vi "add_test.vi"() -> ()   [LabVIEW 2018]
panel:
  in  "Input Parameters":string
  out "Current Pressure [Torr]":dbl
  out "Average Pressure [Torr]":dbl
  out "Average Press.  < 2.2E-4 Torr?":bool
  in  "Run Scan?":bool
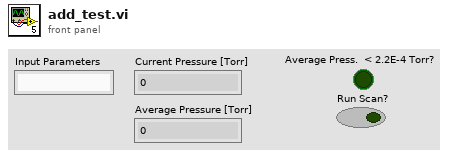
[diagram p1: front panel]
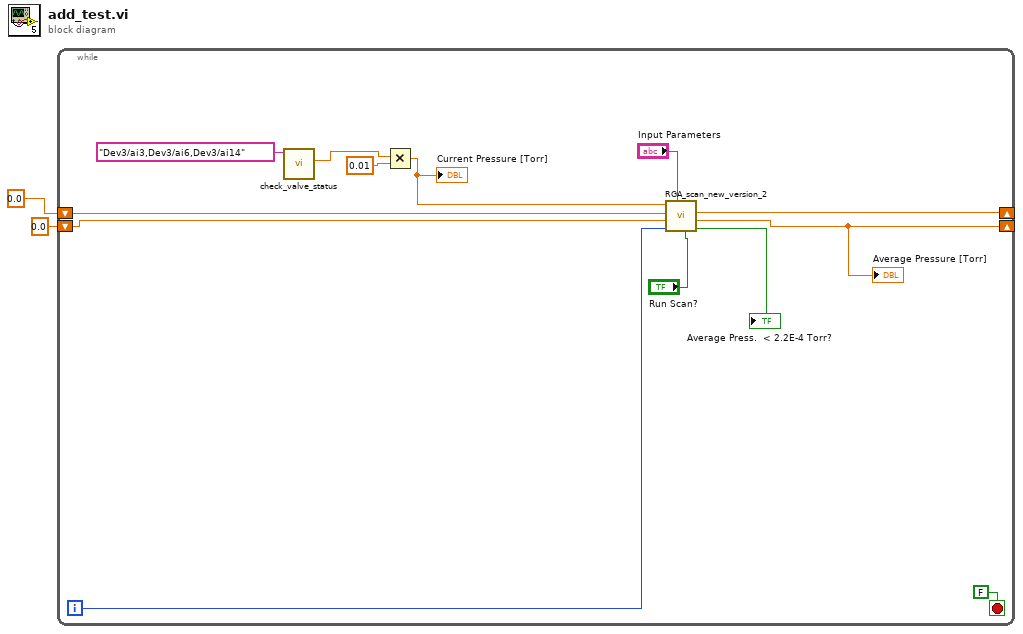
[diagram p0: block diagram]
diagram:
  n1 = while {
    shift-right: [w10] -> _
    shift-left: 0.0 ("Running Sum") -> [w7]
    shift-right: [w9] -> _
    shift-left: 0.0 ("Running Average") -> [w8]
    i -> [w11]
    stop <- FALSE ("stop") stop-if-true
    n2 = call "check_valve_status.vi"("Channel 1"=tag "Dev3/ai3,Dev3/ai6,Dev3/ai14") -> ("Ch. 2 value"=w14:dbl)  [unwired: 8 in, 2 out]
    n3 = Multiply(x=w14, y=0.01) -> (x*y=w13:dbl)
    "Current Pressure [Torr]" <- w13
    n4 = call "RGA_scan_new_version_2.vi"("Run Scan?"="Run Scan?", "Input Parameters"="Input Parameters", "Current Iteration"=w11, "Previous Loop Avg."=w8, "Previous Loop Sum"=w7, "Current Pressure Reading"=w13) -> ("Average Press.  < 2.2E-4 Torr?"=→"Average Press.  < 2.2E-4 Torr?":bool, "Running Average"=w9:dbl, "Running Sum"=w10:dbl)  [unwired: 3 in]
    "Average Pressure [Torr]" <- w9
  }
